vi "NI-DCPower Source DC Voltage.vi"(0 "Resource Name":refnum<k15>="Dev1", 2 "Channel Name":string="0", 3 "Voltage Level":dbl=2.0 format="%_6p", 4 "Current Limit":dbl=0.1 format="%_6p", 5 "Source Delay (Sec)":dbl=0.1 format="%_6p", 6 "Voltage Level Range":dbl=6.0 format="%_6p", 8 "Current Limit Range":dbl=0.1 format="%_6p") -> (15 "Voltage Measurement":dbl, 16 "Current Measurement":dbl, 17 "Compliance/Limit Reached":bool)   [LabVIEW 2014]
doc: "Demonstrates how to use the DC Voltage Output Function to force an output voltage. This example initializes a session, configures the Output Function, Sense, Autorange, Voltage Level and Current Limit, initiates generation, waits for a specified delay, and measures the voltage and current output. This example uses Single Point source mode."
uses:
  <instrlib>/niDCPower/nidcpower.llb/niDCPower Output Function.ctl
  <instrlib>/niDCPower/nidcpower.llb/niDCPower Source Mode.ctl
  <instrlib>/niDCPower/nidcpower.llb/niDCPower Wait For Event - Event.ctl
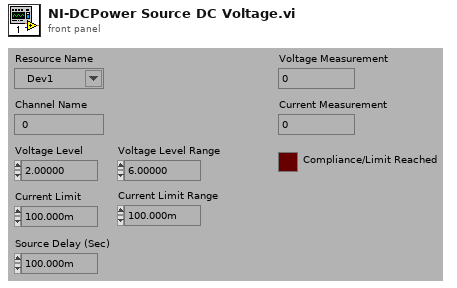
[diagram p1: front panel]
types:
  T1 = typedef "niDCPower Wait For Event - Event.ctl" = i32
  T2 = typedef "niDCPower Source Mode.ctl" = i32
  T3 = typedef "niDCPower Output Function.ctl" = i32
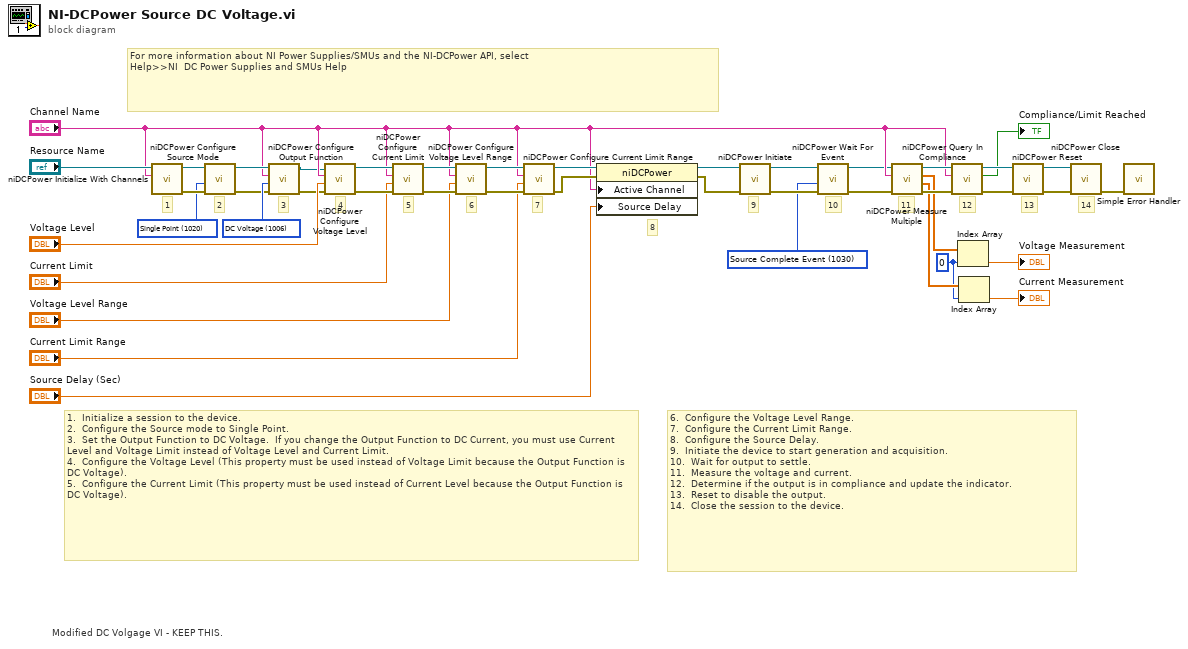
[diagram p0: block diagram]
diagram:
  w4 = T1 1030 items=["Source Complete Event"=1030, "Measure Complete Event"=1031, "Sequence Iteration Complete Event"=1032, "Sequence Engine Done Event"=1033] ("event")
  w17 = 0 ("index")
  w28 = T2 1020 items=["Single Point"=1020, "Sequence"=1021] ("source mode")
  w33 = T3 1006 items=["DC Voltage"=1006, "DC Current"=1007] ("output function")
  # "Modified DC Volgage VI - KEEP THIS."
  # "For more information about NI Power Supplies/SMUs and the NI-DCPower API, select\nHelp>>NI  DC Power Supplies and SMUs Help"
  # "14"
  # "9"
  # "11"
  # "10"
  # "7"
  # "6"
  # "2"
  # "1.  Initialize a session to the device.\n2.  Configure the Source mode to Single Point.\n3.  Set the Output Function to DC Voltage.  If you change the Output Function to DC Current, you must use Current Level and Voltage Limit instead of Voltage Level and Current Limit.\n4.  Configure the Voltage Level (This property must be used instead of Voltage Limit because the Output Function is DC Voltage).\n5.  Configure the Current Limit (This property must be used instead of Current Level because the Output Function is DC Voltage)."
  # "3"
  # "12"
  # "6.  Configure the Voltage Level Range.\n7.  Configure the Current Limit Range.\n8.  Configure the Source Delay.\n9.  Initiate the device to start generation and acquisition.\n10.  Wait for output to settle.\n11.  Measure the voltage and current.\n12.  Determine if the output is in compliance and update the indicator.\n13.  Reset to disable the output.\n14.  Close the session to the device."
  # "13"
  # "8"
  # "5"
  # "4"
  # "1"
  n1 = call <instrlib>:"niDCPower Initialize With Channels.vi"("channels"="Channel Name", "resource name"="Resource Name") -> ("error out"=w32:errorcluster, "instrument handle out"=w31:refnum<k15>)  [unwired: 3 in, 5 out]
  n2 = call <instrlib>:"niDCPower Configure Source Mode.vi"("error in (no error)"=w32, "source mode"=w28, "instrument handle"=w31) -> ("error out"=w30:errorcluster, "instrument handle out"=w29:refnum<k15>)  [unwired: 7 out]
  n3 = call <instrlib>:"niDCPower Configure Output Function.vi"("error in (no error)"=w30, "output function"=w33, "channel name"="Channel Name", "instrument handle"=w29) -> ("error out"=w2:errorcluster, "instrument handle out"=w3:refnum<k15>)  [unwired: 6 out]
  n4 = call <instrlib>:"niDCPower Configure Voltage Level.vi"("error in (no error)"=w2, "voltage level"="Voltage Level", "channel name"="Channel Name", "instrument handle"=w3) -> ("error out"=w41:errorcluster, "instrument handle out"=w42:refnum<k15>)  [unwired: 6 out]
  n5 = call <instrlib>:"niDCPower Configure Current Limit.vi"("error in (no error)"=w41, "current limit"="Current Limit", "channel name"="Channel Name", "instrument handle"=w42) -> ("error out"=w27:errorcluster, "instrument handle out"=w26:refnum<k15>)  [unwired: 1 in, 5 out]
  n6 = call <instrlib>:"niDCPower Configure Voltage Level Range.vi"("error in (no error)"=w27, "voltage level range"="Voltage Level Range", "channel name"="Channel Name", "instrument handle"=w26) -> ("error out"=w25:errorcluster, "instrument handle out"=w24:refnum<k15>)  [unwired: 6 out]
  n7 = call <instrlib>:"niDCPower Configure Current Limit Range.vi"("error in (no error)"=w25, "current limit range"="Current Limit Range", "channel name"="Channel Name", "instrument handle"=w24) -> ("error out"=w11:errorcluster, "instrument handle out"=w14:refnum<k15>)  [unwired: 6 out]
  n8 = property class="niDCPower"(reference=w14, error in=w11, "Active Channel"="Channel Name", "Source Delay"="Source Delay (Sec)") -> (reference out=w13:refnum<k15>, error out=w12:errorcluster)
  n9 = call <instrlib>:"niDCPower Initiate.vi"("error in (no error)"=w12, "instrument handle"=w13) -> ("error out"=w6:errorcluster, "instrument handle out"=w8:refnum<k15>)  [unwired: 2 in, 6 out]
  n10 = call <instrlib>:"niDCPower Wait For Event.vi"("error in (no error)"=w6, "event"=w4, "instrument handle"=w8) -> ("error out"=w5:errorcluster, "instrument handle out"=w7:refnum<k15>)  [unwired: 1 in, 6 out]
  n11 = call <instrlib>:"niDCPower Measure Multiple.vi"("error in (no error)"=w5, "channel name"="Channel Name", "instrument handle"=w7) -> ("error out"=w20:errorcluster, "current measurements"=w18:dbl[], "voltage measurements"=w19:dbl[], "instrument handle out"=w21:refnum<k15>)  [unwired: 5 out]
  n12 = call <instrlib>:"niDCPower Query In Compliance.vi"("error in (no error)"=w20, "channel name"="Channel Name", "instrument handle"=w21) -> ("error out"=w36:errorcluster, "in compliance?"=→"Compliance/Limit Reached":bool, "instrument handle out"=w39:refnum<k15>)  [unwired: 6 out]
  n13 = Index Array(array=w19, index=w17) -> (element=→"Voltage Measurement":dbl)
  n14 = Index Array(array=w18, index=w17) -> (element=→"Current Measurement":dbl)
  n15 = call <instrlib>:"niDCPower Reset.vi"("error in (no error)"=w36, "instrument handle"=w39) -> ("error out"=w37:errorcluster, "instrument handle out"=w38:refnum<k15>)  [unwired: 2 in, 6 out]
  n16 = call <instrlib>:"niDCPower Close.vi"("error in (no error)"=w37, "instrument handle"=w38) -> ("error out"=w35:errorcluster)  [unwired: 9 out]
  n17 = call <vilib>:"Simple Error Handler.vi"("error in (no error)"=w35) -> ()  [unwired: 1 in, 8 out]
